vi "GEA2 Script Test Automated.vi"(0 "GEA2 Reference In":refnum<k24>, 2 "Test Case":T1, 5 "Standalone":bool, 11 "Error In":errorcluster) -> (4 "GEA2 Reference Out":refnum<k24>, 6 "Pass/Fail?":bool, 8 "Report Text":string, 15 "Error Out":errorcluster)   [LabVIEW 2016]
doc: "This VI measures the time between the double line break closing and a burner relay closing."
uses:
  typedefs/Script Output.ctl
  typedefs/Command Type.ctl
  Q:/Common/DLLs/GEA3/GeaCommunication.dll
  DLLs/GEA3/GeaCommunication.dll
  LabVIEW GEA2 Toolkit/LabVIEW_GEA2_Toolkit.lvlibp/type defs/Data Out.ctl
  LabVIEW GEA2 Toolkit/LabVIEW_GEA2_Toolkit.lvlibp
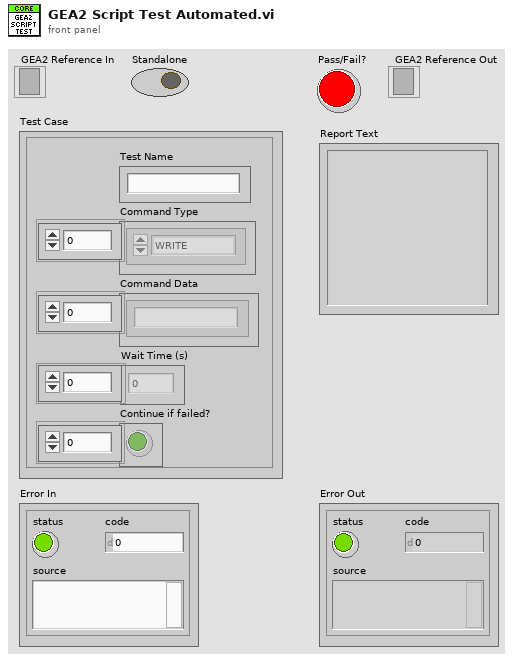
[diagram p1: front panel]
types:
  T1 = typedef "Script Output.ctl" = cluster{"Command Data":string[], "Command Type":T2[], "Test Name":string, "Wait Time (s)":dbl[], "Continue if failed?":bool[]}
  T2 = typedef "Command Type.ctl" = enum16{"WRITE", "READ", "ERDWRITE", "ERDREAD"}
  T3 = typedef "LabVIEW_GEA2_Toolkit.lvlibp/Data Out.ctl" = cluster{"Source":u8, "Destination":u8, "Command":u8, "Length":u8, "CRC":u16, "Message":string}
  T4 = typedef "LabVIEW_GEA2_Toolkit.lvlibp/Data In.ctl" = cluster{"Source":u8, "Destination":u8, "Command":u8, "Message":string}
  T5 = typedef "LabVIEW_GEA2_Toolkit.lvlibp/Source_Destination.ctl" = cluster{"Source":u8, "Destination":u8}
  T6 = typedef "LabVIEW_GEA2_Toolkit.lvlibp/ERD Write Data In.ctl" = cluster{"ERD Number":u16, "Data Type":T7, "Data":string}
  T7 = typedef "LabVIEW_GEA2_Toolkit.lvlibp/Data Type.ctl" = enum16{"string", "boolean", "uint8_t", "uint16_t", "uint32_t", "uint64_t", "int8_t", "int16_t", "int32_t", "int64_t"}
  T8 = typedef "LabVIEW_GEA2_Toolkit.lvlibp/ERD Read Data In.ctl" = cluster{"ERD Number":u16, "Data Type":T7}
  T9 = typedef "LabVIEW_GEA2_Toolkit.lvlibp/ERD Read Data Out.ctl" = cluster{"ERD Number":u16, "Data":string}
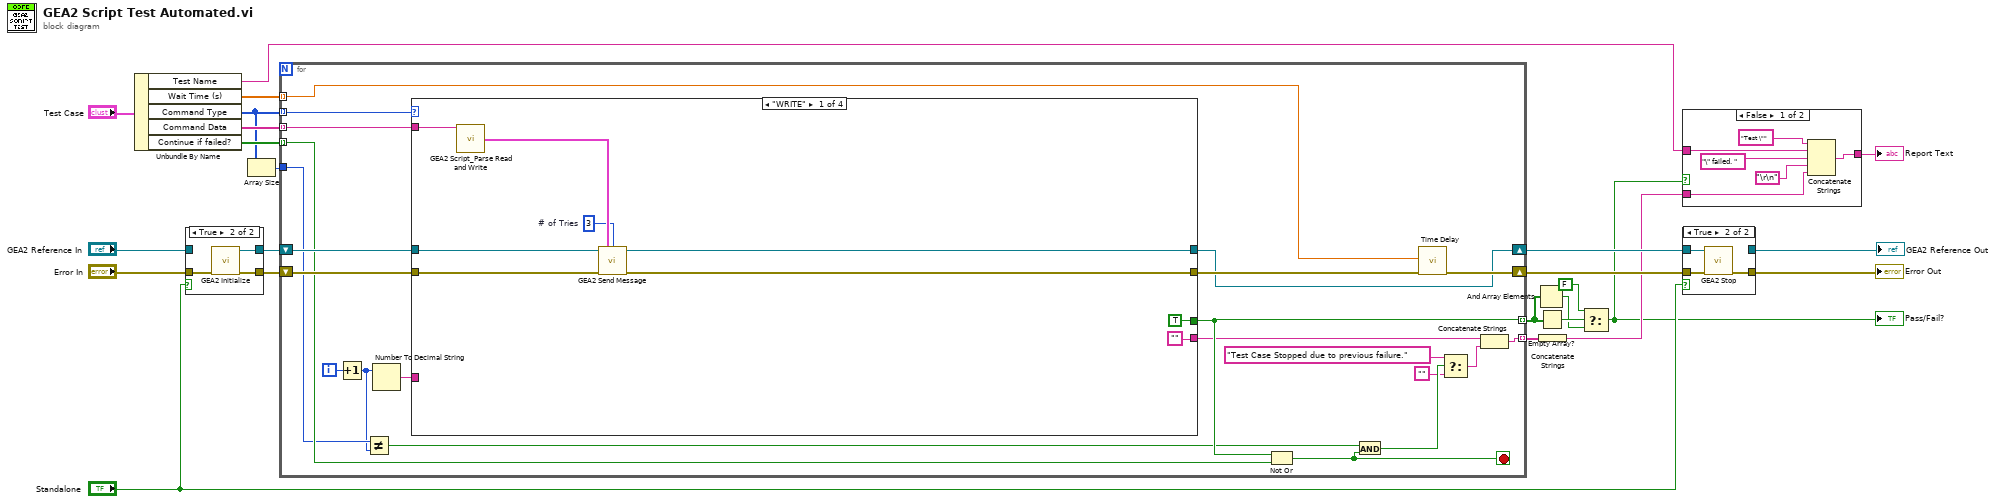
[diagram p0: block diagram]
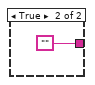
[diagram p2: hidden frame]
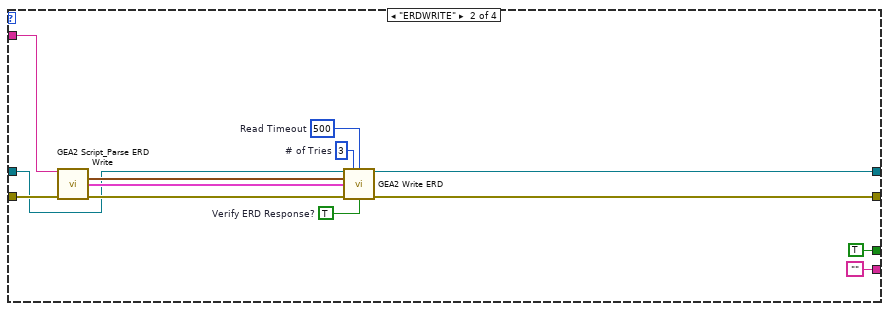
[diagram p3: hidden frame]
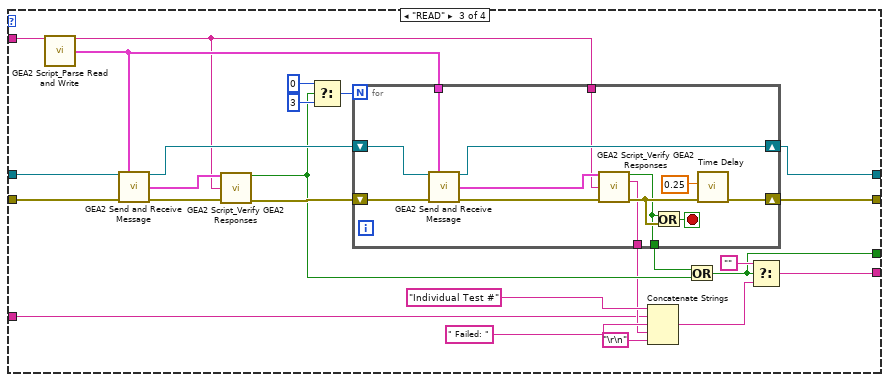
[diagram p4: hidden frame]
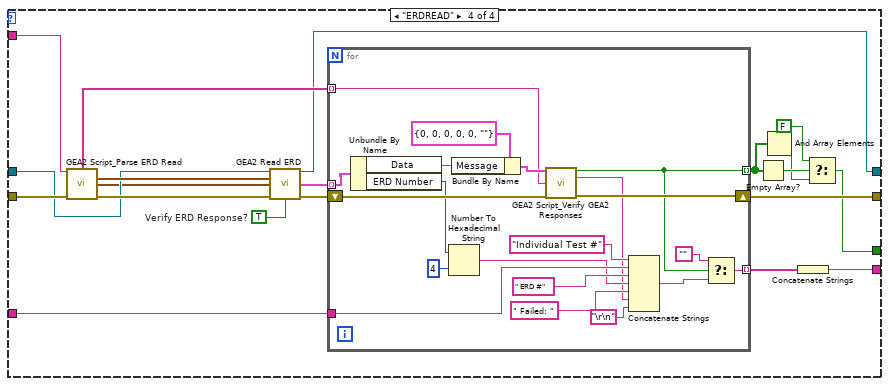
[diagram p5: hidden frame]
diagram:
  n1 = Unbundle By Name("Test Case") -> ("Test Name"=w17:string, "Wait Time (s)"=w16:dbl[], "Command Type"=w2:T2[], "Command Data"=w18:string[], "Continue if failed?"=w11:bool[])
  n2 = case shown="True" "Standalone" {
    tunnel: [w25 w29] -> w20
    tunnel: "GEA2 Reference In" -> [w26 _]
    tunnel: [w26 w27] -> w19
    tunnel: "Error In" -> [w25 w28]
    frame False {
    }
    frame True {
      n3 = call "GEA2 Initialize.vi"("error in"=w28) -> ("GEA2 Reference Out"=w27:refnum<k24>, "error out"=w29:errorcluster)  [unwired: 12 in, 1 out]
    }
  }
  n4 = Array Size(array=w2) -> (size(s)=w1:i32)
  n5 = for {
    shift-right: [w51] -> w14
    shift-left: w20 -> [w49]
    shift-right: [w44] -> w13
    shift-left: w19 -> [w48]
    tunnel: w2 -> [w50] mode=indexing
    tunnel: w18 -> [w47] mode=indexing
    tunnel: w16 -> [w45] mode=indexing
    tunnel: w11 -> [w43] mode=indexing
    tunnel: [w38] -> w10 mode=indexing
    tunnel: [w42] -> w6 mode=indexing
    tunnel: w1 -> [w36]
    i -> [w41]
    stop <- w33 stop-if-true
    n6 = Increment(x=w41) -> (x+1=w35:i32)
    n7 = Not Equal?(x=w36, y=w35) -> (x != y?=w34:bool)
    n8 = Number To Decimal String(number=w35) -> (decimal integer string=w40:string)  [unwired: 1 in]
    n9 = case shown="\"WRITE\"" w50 {
      tunnel: w49 -> [w59 w68 w97 w130]
      tunnel: w48 -> [w58 w64 w96 w127]
      tunnel: w47 -> [w60 w69 w98 w126]
      tunnel: [w56 w72 w87 w124] -> w46
      tunnel: [w57 w73 w88 w120] -> w44
      tunnel: w40 -> [_ _ w74 w112]
      tunnel: ["" "" w78 w118] -> w39
      tunnel: [TRUE ("t") TRUE ("t") w75 w113] -> w42
      frame "WRITE" {
        w52 = u8 3  # # of Tries
        n10 = call "GEA2 Script_Parse Read and Write.vi"("Data"=w60) -> ("GEA2 Message"=w55:T4)  [unwired: 13 in, 1 out]
        n11 = call "GEA2 Send Message.vi"("GEA2 Reference In"=w58, "Input Data"=w55, "# of Tries"=w52, "Error In"=w59) -> ("GEA2 Reference Out"=w57:refnum<k24>, "Error Out"=w56:errorcluster)  [unwired: 10 in]
      }
      frame "ERDWRITE" {
        w61 = u8 3  # # of Tries
        w70 = TRUE  # Verify ERD Response?
        w71 = u32 500  # Read Timeout
        n12 = call "GEA2 Script_Parse ERD Write.vi"("Data"=w69, "Error In"=w68) -> ("GEA Inputs"=w65:T5, "Write ERD List"=w66:T6[], "Error Out"=w67:errorcluster)  [unwired: 11 in]
        n13 = call "GEA2 Write ERD.vi"("GEA2 Reference In"=w64, "# of Tries"=w61, "Read Timeout (ms)"=w71, "GEA Inputs"=w65, "Write ERD List"=w66, "Error In"=w67, "Verify ERD Response?"=w70) -> ("GEA2 Reference Out"=w73:refnum<k24>, "Error Out"=w72:errorcluster)  [unwired: 6 in, 1 out]
      }
      frame "READ" {
        n14 = call "GEA2 Script_Parse Read and Write.vi"("Data"=w98) -> ("Expected Response"=w76:string, "GEA2 Message"=w77:T4)  [unwired: 13 in]
        n15 = call "GEA2 Send and Receive Message.vi"("GEA2 Reference In"=w96, "Input Data"=w77, "Error In"=w97) -> ("GEA2 Reference Out"=w92:refnum<k24>, "Converted Data Out"=w95:T3, "Error Out"=w94:errorcluster)  [unwired: 9 in, 1 out]
        n16 = call "GEA2 Script_Verify GEA2 Responses.vi"("Actual Response"=w95, "Expected Response"=w76, "Error In"=w94) -> ("Pass/Fail?"=w85:bool, "Error Out"=w93:errorcluster)  [unwired: 10 in, 1 out]
        n17 = Select(t=0, s=w85, f=3) -> (s? t:f=w89:i32)
        n18 = for {
          N: w89 -> [_]
          shift-right: [w107] -> w87
          shift-left: w93 -> [w110]
          shift-right: [w108] -> w88
          shift-left: w92 -> [w109]
          tunnel: w76 -> [w103]
          tunnel: [w101] -> w81
          tunnel: w77 -> [w100]
          tunnel: [w99] -> w86
          stop <- w111 stop-if-true
          n19 = call "GEA2 Send and Receive Message.vi"("GEA2 Reference In"=w109, "Input Data"=w100, "Error In"=w110) -> ("GEA2 Reference Out"=w108:refnum<k24>, "Converted Data Out"=w104:T3, "Error Out"=w105:errorcluster)  [unwired: 9 in, 1 out]
          n20 = call "GEA2 Script_Verify GEA2 Responses.vi"("Actual Response"=w104, "Expected Response"=w103, "Error In"=w105) -> ("Pass/Fail?"=w99:bool, "Report Text"=w101:string, "Error Out"=w102:errorcluster)  [unwired: 10 in]
          n21 = Or(x=w99, y=w102) -> (x .or. y?=w111:bool)
          n22 = call "Time Delay"("error in (no error)"=w102, "Delay Time (s)"=0.25) -> ("error out"=w107:errorcluster)  [unwired: 9 in]
        }
        n23 = Concatenate Strings("Individual Test #", w74, " Failed: " ("string"), w81, "\r\n") -> (w79:string)
        n24 = Or(x=w86, y=w85) -> (x .or. y?=w75:bool)
        n25 = Select(t="", s=w75, f=w79) -> (s? t:f=w78:string)
      }
      frame "ERDREAD" {
        w131 = TRUE  # Verify ERD Response?
        n26 = call "GEA2 Script_Parse ERD Read.vi"("Data"=w126, "Error In"=w130) -> ("Expected Responses"=w122:string[], "GEA Inputs"=w128:T5, "Read ERD List"=w121:T8[], "Error Out"=w129:errorcluster)  [unwired: 10 in]
        n27 = call "GEA2 Read ERD.vi"("GEA2 Reference In"=w127, "GEA Inputs"=w128, "Read ERD List"=w121, "Error In"=w129, "Verify ERD Response?"=w131) -> ("GEA2 Reference Out"=w120:refnum<k24>, "ERD Data Out"=w123:T9[], "Error Out"=w125:errorcluster)  [unwired: 7 in, 1 out]
        n28 = for {
          shift-right: [w145] -> w124
          shift-left: w125 -> [w148]
          tunnel: w123 -> [w151] mode=indexing
          tunnel: w122 -> [w146] mode=indexing
          tunnel: [w135] -> w117 mode=indexing
          tunnel: w112 -> [w139]
          tunnel: [w134] -> w119 mode=indexing
          n29 = Unbundle By Name(w151) -> ("Data"=w147:string, "ERD Number"=w142:u16)
          n30 = Number To Hexadecimal String(1:i16 4 ("width (-)"), 2:w142) -> (0:w137:string)
          n31 = Bundle By Name(cluster=T3 {"Source"=0, "Destination"=0, "Command"=0, "Length"=0, "CRC"=0, "Message"=""} ("Actual Response"), "Message"=w147) -> (w149:T3)
          n32 = call "GEA2 Script_Verify GEA2 Responses.vi"("Actual Response"=w149, "Expected Response"=w146, "Error In"=w148) -> ("Pass/Fail?"=w135:bool, "Report Text"=w133:string, "Error Out"=w145:errorcluster)  [unwired: 10 in]
          n33 = Concatenate Strings("Individual Test #", w139, " ERD #", w137, " Failed: " ("string"), w133, "\r\n") -> (w144:string)
          n34 = Select(t="", s=w135, f=w144) -> (s? t:f=w134:string)
        }
        n35 = Empty Array?(array=w117) -> (empty?=w116:bool)
        n36 = And Array Elements(Boolean array=w117) -> (logical AND=w115:bool)
        n37 = Concatenate Strings(w119) -> (w118:string)
        n38 = Select(t=FALSE, s=w116, f=w115) -> (s? t:f=w113:bool)
      }
    }
    n39 = Not Or(1:w43, 2:w42) -> (0:w33:bool)
    n40 = And(x=w34, y=w33) -> (x .and. y?=w31:bool)
    n41 = call "Time Delay"("error in (no error)"=w46, "Delay Time (s)"=w45) -> ("error out"=w51:errorcluster)  [unwired: 9 in]
    n42 = Select(t="Test Case Stopped due to previous failure." ("f"), s=w31, f="") -> (s? t:f=w37:string)
    n43 = Concatenate Strings(w39, w37) -> (w38:string)
  }
  n44 = And Array Elements(Boolean array=w6) -> (logical AND=w8:bool)
  n45 = Empty Array?(array=w6) -> (empty?=w9:bool)
  n46 = Concatenate Strings(w10) -> (w5:string)
  n47 = Select(t=FALSE, s=w9, f=w8) -> (s? t:f=w4:bool)
  "Pass/Fail?" <- w4
  n48 = case shown="False" w4 {
    tunnel: w17 -> [w156 _]
    tunnel: [w154 ""] -> w22
    tunnel: w5 -> [w153 _]
    frame False {
      n49 = Concatenate Strings("Test \"", w156, "\" failed. " ("string"), "\r\n", w153) -> (w154:string)
    }
    frame True {
    }
  }
  "Report Text" <- w22
  n50 = case shown="True" "Standalone" {
    tunnel: [w160 w163] -> w12
    tunnel: w14 -> [w160 w162]
    tunnel: w13 -> [w159 w161]
    tunnel: [w159 _] -> w3
    frame False {
    }
    frame True {
      n51 = call "GEA2 Stop.vi"("GEA2 Reference In"=w161, "Error In"=w162) -> ("Error Out"=w163:errorcluster)  [unwired: 13 in]
    }
  }
  "Error Out" <- w12
  "GEA2 Reference Out" <- w3
